vi "while.vi"() -> ()   [LabVIEW 2020]
panel:
  out "Array":i32[](array[numeric])
  out "Numeric":i32
  in  "stop":bool
  # "while(1){\n\n\n}"
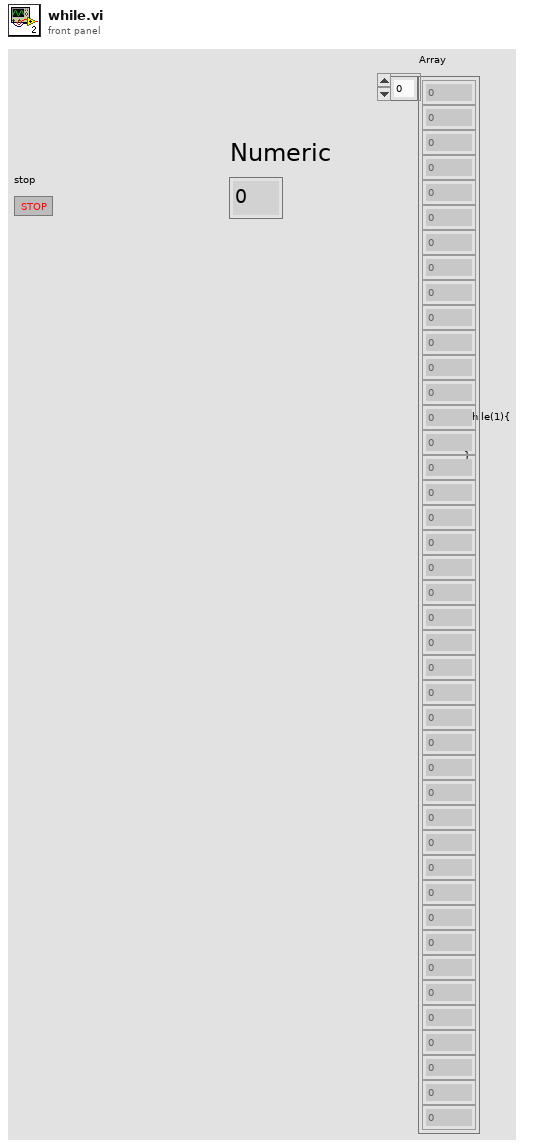
[diagram p1: front panel]
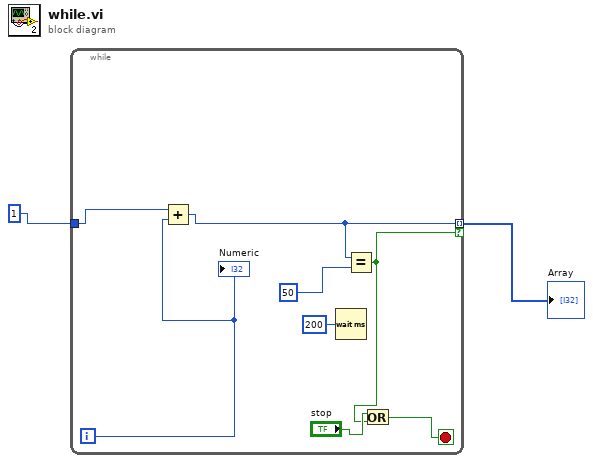
[diagram p0: block diagram]
diagram:
  n1 = while {
    tunnel: 1 -> [w4]
    tunnel: [w7] -> w1 mode=indexing if=w3
    i -> [w9]
    stop <- w5 stop-if-true
    n2 = Add(x=w4, y=w9) -> (x+y=w7:i32)
    n3 = Wait (ms)(milliseconds to wait=u32 200) -> ()  [unwired: 1 out]
    n4 = Equal?(x=w7, y=50) -> (x = y?=w3:bool)
    n5 = Or(x="stop", y=w3) -> (x .or. y?=w5:bool)
    "Numeric" <- w9
  }
  "Array" <- w1
